vi "CreateWorkflowAndConfigFiles.vi"(8 "error in (no error)":errorcluster, 11 "Repo Folder Path":path=path "C:/sw-deps-monitor/Source") -> (0 "error out":errorcluster, 1 "Confi File path":path, 2 "CICD Config Created?":bool, 3 "Workflow File Created?":bool, 5 "New YAML Files":path[](array[path]))   [LabVIEW 2023, in "DepsWatchToolsMenu.lvlib"]
uses:
  DepsWatchToolsMenu.lvlib
  <userlib>/_OpenG.lib/file/file.llb/openg_file.lvlib
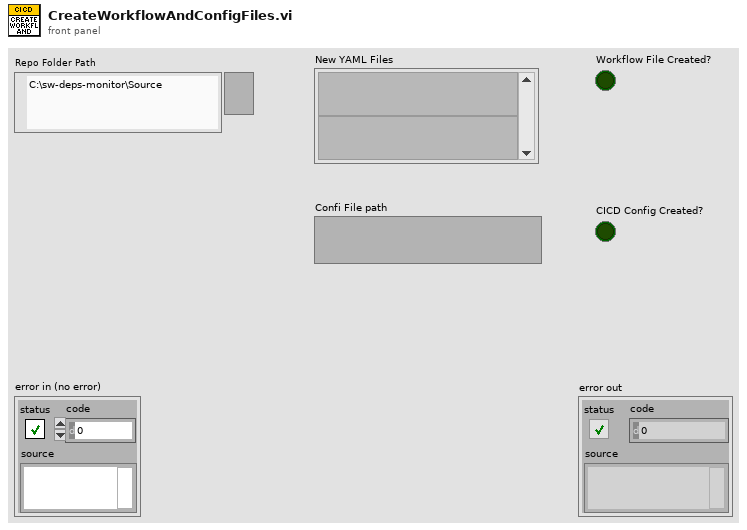
[diagram p1: front panel]
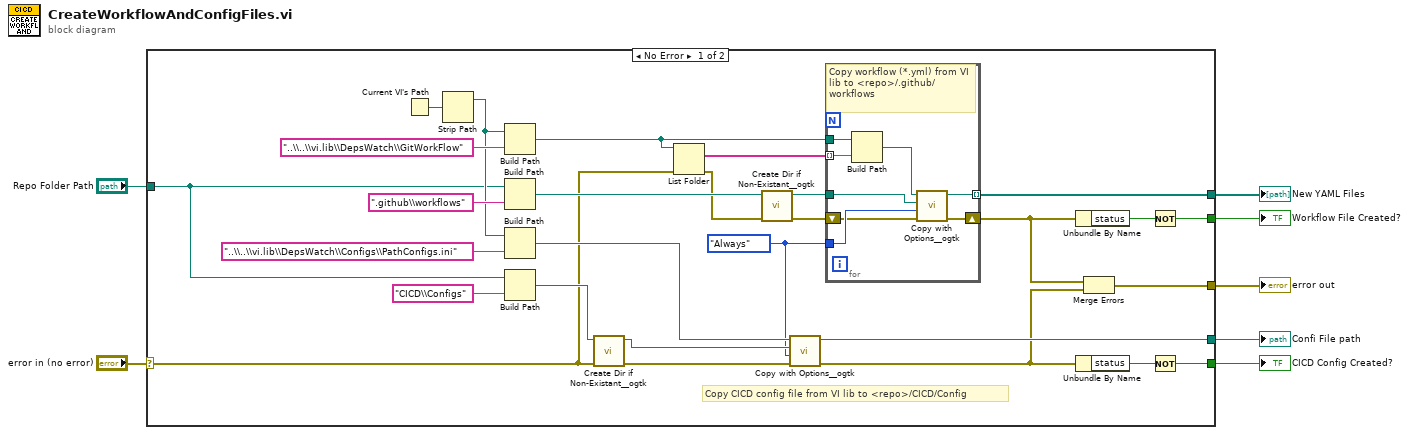
[diagram p0: block diagram]
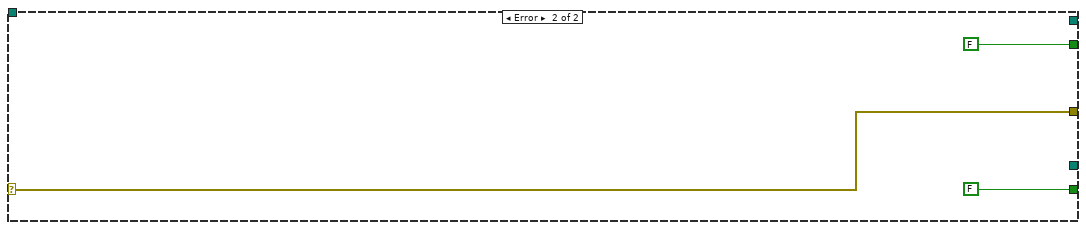
[diagram p2: hidden frame]
diagram:
  n1 = case shown="No Error" "error in (no error)" {
    selector: "error in (no error)" -> [w8 w45]
    tunnel: [w31 _] -> w7
    tunnel: [w20 _] -> w6
    tunnel: [w18 FALSE] -> w5
    tunnel: [w15 FALSE] -> w4
    tunnel: [w14 w45] -> w3
    tunnel: "Repo Folder Path" -> [w11 _]
    frame No Error {
      w21 = enum16{"Never", "Always", "If Newer"}."Always" ("Replace Mode (Never)")
      # "Copy CICD config file from VI lib to <repo>/CICD/Config"
      n2 = Current VI's Path() -> (path=w35:path)
      n3 = Strip Path(path=w35) -> (stripped path=w12:path)  [unwired: 1 out]
      n4 = Build Path(base path=w12, name or relative path="..\\..\\vi.lib\\DepsWatch\\GitWorkFlow") -> (appended path=w28:path)
      n5 = Build Path(base path=w11, name or relative path=".github\\workflows") -> (appended path=w32:path)
      n6 = Build Path(base path=w12, name or relative path="..\\..\\vi.lib\\DepsWatch\\Configs\\PathConfigs.ini") -> (appended path=w22:path)
      n7 = Build Path(base path=w11, name or relative path="CICD\\Configs") -> (appended path=w24:path)
      n8 = call <userlib>:"Create Dir if Non-Existant__ogtk.vi"("error in (no error)"=w8, "Directory Path"=w24) -> ("error out"=w10:errorcluster, "dup Directory Path"=w23:path)  [unwired: 7 in, 1 out]
      n9 = List Folder(path=w28, error in=w8) -> (filenames=w27:string[], error out=w9:errorcluster)  [unwired: 2 in, 2 out]
      n10 = call <userlib>:"Create Dir if Non-Existant__ogtk.vi"("error in (no error)"=w9, "Directory Path"=w32) -> ("error out"=w29:errorcluster, "dup Directory Path"=w30:path)  [unwired: 7 in, 1 out]
      n11 = call <userlib>:"Copy with Options__ogtk.vi"("error in (no error)"=w10, "Replace Mode (Never)"=w21, "target path"=w23, "source path"=w22) -> ("error out"=w13:errorcluster, "new path"=w20:path)  [unwired: 6 in]
      n12 = for {
        tunnel: w21 -> [w43]
        tunnel: w30 -> [w40]
        shift-right: [w41] -> w17
        shift-left: w29 -> [w39]
        tunnel: w28 -> [w38]
        tunnel: [w42] -> w31 mode=indexing
        tunnel: w27 -> [w37] mode=indexing
        # "Copy workflow (*.yml) from VI lib to <repo>/.github/workflows"
        n13 = Build Path(base path=w38, name or relative path=w37) -> (appended path=w36:path)
        n14 = call <userlib>:"Copy with Options__ogtk.vi"("error in (no error)"=w39, "Replace Mode (Never)"=w43, "target path"=w40, "source path"=w36) -> ("error out"=w41:errorcluster, "new path"=w42:path)  [unwired: 6 in]
      }
      n15 = Unbundle By Name(w17) -> ("status"=w16:bool)
      n16 = Unbundle By Name(w13) -> ("status"=w19:bool)
      n17 = Merge Errors(w17, w13) -> (w14:errorcluster)
      n18 = Not(x=w16) -> (.not. x?=w15:bool)
      n19 = Not(x=w19) -> (.not. x?=w18:bool)
    }
    frame Error {
    }
  }
  "error out" <- w3
  "Workflow File Created?" <- w4
  "CICD Config Created?" <- w5
  "New YAML Files" <- w7
  "Confi File path" <- w6
